vi "LAC Cmd_Excution.vi"(7 "timeout(ms)":u32, 8 "error in":errorcluster, 10 "Cmd_exec":T1 items=["Stop meas.", "Start meas.", "Auto-adj. LD output", "Zero reset", "Zero set", "OFFSETTILT judge 1", "OFFSETTILT judge 2"], 11 "VISA name in":refnum<visa-resource-name>) -> (0 "error out":errorcluster, 1 "read buffer":string, 3 "VISA name out":refnum<visa-resource-name>)   [LabVIEW 8.6]
uses:
  TypeDef/H410 Cmd_exec TypeDef.ctl
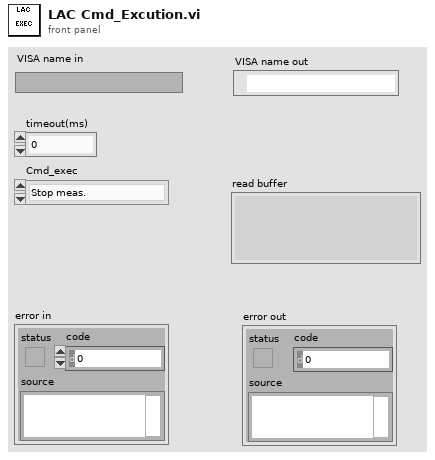
[diagram p1: front panel]
types:
  T1 = typedef "H410 Cmd_exec TypeDef.ctl" = u16
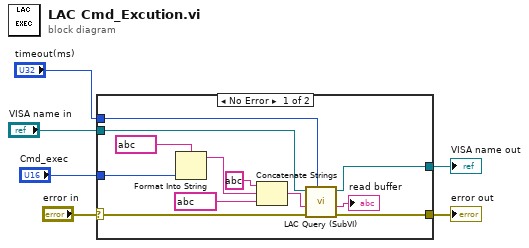
[diagram p0: block diagram]
diagram:
  n1 = case shown="No Error" "error in" {
    selector: "error in" -> [w13 w20]
    tunnel: "VISA name in" -> [w15 w19]
    tunnel: [w18 w19] -> w5
    tunnel: [w16 w20] -> w4
    tunnel: "timeout(ms)" -> [w14 _]
    tunnel: "Cmd_exec" -> [w9 _]
    frame #0 {
      n2 = Format Into String(format string=string ?, w9) -> (resulting string=w7:string)  [unwired: 2 in, 1 out]
      n3 = Concatenate Strings(string ? ("string"), w7, string ? ("write buffer")) -> (w11:string)
      n4 = call "LAC Query (SubVI).vi"("timeout(ms)"=w14, "error in"=w13, "Command"=w11, "VISA name in"=w15) -> ("error out"=w16:errorcluster, "read buffer"=→"read buffer":string, "VISA name out"=w18:refnum<visa-resource-name>)  [unwired: 5 in]
    }
    frame #1 {
    }
  }
  "VISA name out" <- w5
  "error out" <- w4
